vi "DB Update array data(cmd).vi"(7 "Data":string[](array[string]), 8 "error in (no error)":errorcluster caption="错误输入（无错误）", 9 "columns":string[](array[string]), 10 "table name":string, 11 "Connncet State":T2) -> (0 "error out":errorcluster caption="错误输出", 2 "connection reference":T1, 3 "Connncet State out":T2)   [LabVIEW 2014]
uses:
  <vilib>/addons/database/NI_Database_API.lvlib
  <vilib>/addons/database/Connection.llb/Conn Execute.vi
  <vilib>/addons/database/Recordset.llb/Rec Destroy - Connection.vi
  Ctr/Constr.ctl
  <vilib>/addons/database/Connection.llb/Conn ObjectReference.ctl
  Ctr/Conneect State.ctl
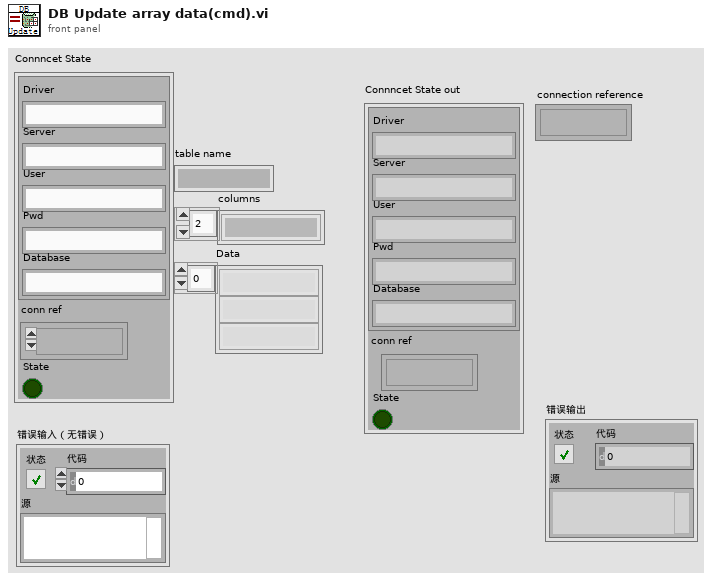
[diagram p1: front panel]
types:
  T1 = typedef "NI_Database_API.lvlib/Conn ObjectReference.ctl" = refnum<k1>
  T2 = typedef "Conneect State.ctl" = cluster{"Constr":T3, "conn ref":T1, "State":bool}
  T3 = typedef "Constr.ctl" = cluster{"Driver":string, "Server":string, "User":string, "Pwd":string, "Database":string}
  T4 = typedef "NI_Database_API.lvlib/Rec ObjectReference.ctl" = refnum<k1>
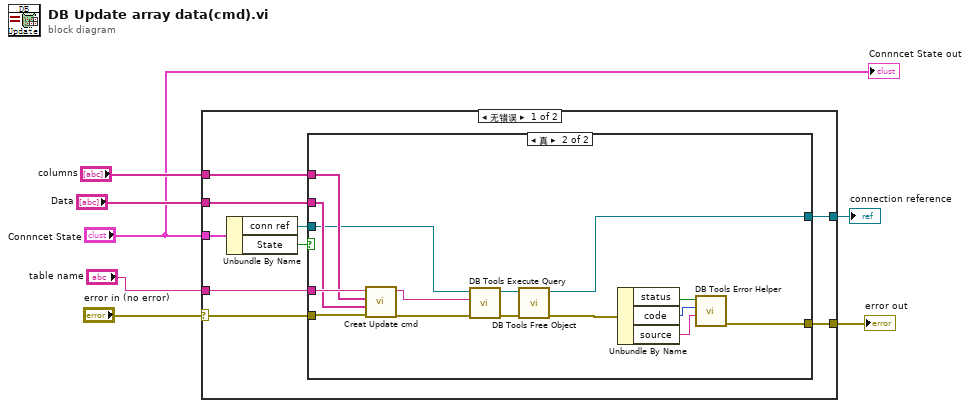
[diagram p0: block diagram]
diagram:
  n1 = case shown="无错误" "error in (no error)" {
    selector: "error in (no error)" -> [w14 w34]
    tunnel: "Connncet State" -> [w16 _]
    tunnel: "table name" -> [w13 _]
    tunnel: "Data" -> [w12 _]
    tunnel: "columns" -> [w11 _]
    tunnel: [w9 w34] -> w3
    tunnel: [w8 _] -> w1
    frame No Error {
      n2 = Unbundle By Name(w16) -> ("conn ref"=w10:T1, "State"=w15:bool)
      n3 = case shown="真" w15 {
        tunnel: w14 -> [w18 w33]
        tunnel: w13 -> [_ w32]
        tunnel: w12 -> [_ w31]
        tunnel: w11 -> [_ w30]
        tunnel: w10 -> [w17 w28]
        tunnel: [w18 w20] -> w9
        tunnel: [w17 w19] -> w8
        frame False {
        }
        frame True {
          n4 = call "Creat Update cmd.vi"("error in (no error)"=w33, "Data"=w31, "columns"=w30, "table name"=w32) -> ("error out"=w29:errorcluster, "insert query"=w27:string)  [unwired: 6 in]
          n5 = call-poly <vilib>:"DB Tools Execute Query.vi"("error in (no error)"=w29, "SQL query"=w27, "connection reference"=w28) -> ("error out"=w23:errorcluster, "recordset reference"=w22:T4)  [unwired: 5 in]
          n6 = call-poly <vilib>:"DB Tools Free Object.vi"("error in (no error)"=w23, "recordset reference"=w22) -> ("error out"=w21:errorcluster, "connection reference"=w19:T1)  [unwired: 8 in]
          n7 = Unbundle By Name(w21) -> ("status"=w24:bool, "code"=w26:i32, "source"=w25:string)
          n8 = call <vilib>:"DB Tools Error Helper.vi"("source"=w25, "code"=w26, "status"=w24) -> ("error out"=w20:errorcluster)  [unwired: 8 in]
        }
      }
    }
    frame Error {
    }
  }
  "error out" <- w3
  "connection reference" <- w1
  "Connncet State out" <- "Connncet State"
